vi "init.vi"(8 "error in (no error)":errorcluster, 11 "ILCTC in":refnum<class "ILCTC.lvclass">) -> (0 "error out":errorcluster, 3 "ILCTC out":refnum<class "ILCTC.lvclass">)   [LabVIEW 2015, in "ILCTC.lvclass"]
uses:
  ILCTC.lvclass
  <userlib>/Common/ILC/Configuration/Serial.ctl
  <userlib>/Common/SerialProtocols/Configuration/SerialConfig.ctl
  <userlib>/Common/SerialProtocols/Configuration/SerialProtocol.ctl
  <userlib>/Common/SerialProtocols/Configuration/ProtocolParameters.ctl
  <userlib>/Common/SerialProtocols/Configuration/SerialMessageParameters.ctl
  <userlib>/Common/ILC/Configuration/ADC Conversion Settings.ctl
  <userlib>/Common/ILC/Configuration/ADC Collection Settings.ctl
  <userlib>/Common/ILC/Typedefs/Input Channels.ctl
  <userlib>/Common/ILC/Typedefs/Scan Rates.ctl
  <userlib>/Common/ILC/Configuration/DAC Settings.ctl
  <userlib>/Common/ILC/ILC/ILC.lvclass/ILC.ctl
  <userlib>/Common/ILC/ILC/ILC.lvclass
  <userlib>/Common/SerialProtocols/SerialProtocols.lvlib
  <userlib>/Common/ILC/Configuration/ILCConfiguration.lvlib
  ConfigurationThisComponent/ConfigurationThisComponent.lvclass
  <userlib>/Common/ILC/Typedefs/ILCTypedefs.lvlib
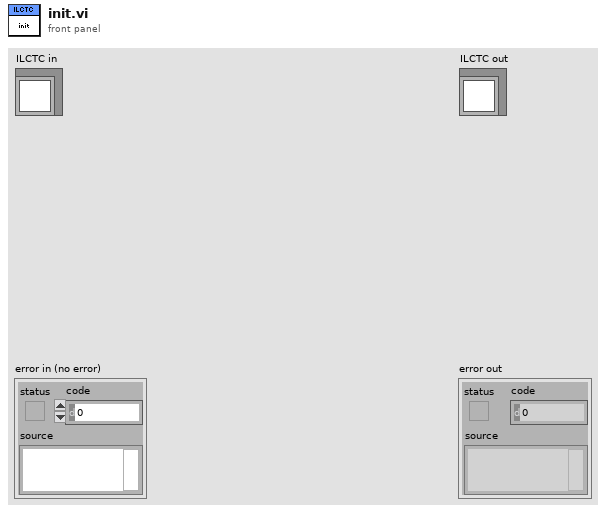
[diagram p1: front panel]
types:
  T1 = typedef "ILCCommon.lvlib/ILCConfiguration.lvlib/DAC Settings.ctl" = cluster{"Voltage Reference":dbl[unit], "Min Counts":i32, "Max Counts":i32}
  T2 = typedef "ILCCommon.lvlib/ILCConfiguration.lvlib/ADC Collection Settings.ctl" = cluster{"Input Channels":T3, "Scan Rate (Hz) ":T4, "PGA Gain Coefficient":u8}
  T3 = typedef "ILCCommon.lvlib/ILCTypedefs.lvlib/Input Channels.ctl" = enum16{"Channel 0", "3 Channels", "5 Channels"}
  T4 = typedef "ILCCommon.lvlib/ILCTypedefs.lvlib/Scan Rates.ctl" = enum16{"50", "60", "100", "120", "200", "240", "300", "400", "480", "600", "1200", "2400", "4800"}
  T5 = typedef "ILCCommon.lvlib/ILCConfiguration.lvlib/ADC Conversion Settings.ctl" = cluster{"Reference Voltage Vref":dbl[unit], "Nominal Input Range in Counts":u32, "Preamplifier Gain (K1 * K2)":dbl, "Conversion Settling Cycles":u16, "Excitation Voltage Vexc":dbl[unit]}
  T6 = typedef "ILCCommon.lvlib/ILCConfiguration.lvlib/Serial.ctl" = cluster{"Serial":T7}
  T7 = typedef "SerialProtocols.lvlib/SerialConfig.ctl" = cluster{"Serial Protocol":T8, "Protocol Parameters":T9, "Serial Message Parameters":T10}
  T8 = typedef "SerialProtocols.lvlib/SerialProtocol.ctl" = enum16{"RS232", "RS485", "SerialSimulator"}
  T9 = typedef "SerialProtocols.lvlib/ProtocolParameters.ctl" = cluster{"VISA resource name":refnum<visa-resource-name>, "Baud Rate":u32, "Data Bits":u16, "Parity":enum16{"None", "Odd", "Even", "Mark", "Space"}, "Flow Control":u16, "Stop Bits":u16, "Timeout (ms)":u32}
  T10 = typedef "SerialProtocols.lvlib/SerialMessageParameters.ctl" = cluster{"Byte Count":u32, "Enable Termination Character":bool, "Termination Char":u8}
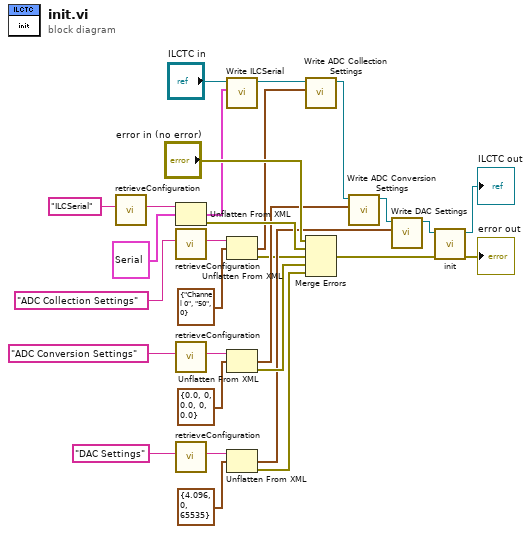
[diagram p0: block diagram]
diagram:
  n1 = call "retrieveConfiguration.vi"("configName"="ILCSerial") -> ("xmlConfig"=w24:string)  [unwired: 8 in, 2 out]
  n2 = Unflatten From XML(xml string=w24, type=T6 {"Serial"={"Serial Protocol"=enum."RS232", "Protocol Parameters"={"VISA resource name"="", "Baud Rate"=0, "Data Bits"=0, "Parity"=enum."None", "Flow Control"=0, "Stop Bits"=0, "Timeout (ms)"=0}, "Serial Message Parameters"={"Byte Count"=0, "Enable Termination Character"=FALSE, "Termination Char"=0}}} ("ILC")) -> (value=w18:T6, error out=w27:errorcluster)  [unwired: 1 in]
  n3 = call "retrieveConfiguration.vi"("configName"="ADC Collection Settings") -> ("xmlConfig"=w4:string)  [unwired: 8 in, 2 out]
  n4 = call "retrieveConfiguration.vi"("configName"="ADC Conversion Settings") -> ("xmlConfig"=w22:string)  [unwired: 8 in, 2 out]
  n5 = call "retrieveConfiguration.vi"("configName"="DAC Settings") -> ("xmlConfig"=w8:string)  [unwired: 8 in, 2 out]
  n6 = call <userlib>:"Write ILCSerial.vi"("ILC Serial"=w18, "ILC in"="ILCTC in") -> ("ILC out"=w12:refnum<class "ILCTC.lvclass">)  [unwired: 9 in]
  n7 = Unflatten From XML(xml string=w4, type=T2 {"Input Channels"=enum."Channel 0", "Scan Rate (Hz) "=enum."50", "PGA Gain Coefficient"=0} ("ADC Collection Settings")) -> (value=w2:T2, error out=w1:errorcluster)  [unwired: 1 in]
  n8 = Unflatten From XML(xml string=w22, type=T5 {"Reference Voltage Vref"=0.0, "Nominal Input Range in Counts"=0, "Preamplifier Gain (K1 * K2)"=0.0, "Conversion Settling Cycles"=0, "Excitation Voltage Vexc"=0.0} ("ILC ADC")) -> (value=w17:T5, error out=w21:errorcluster)  [unwired: 1 in]
  n9 = Unflatten From XML(xml string=w8, type=T1 {"Voltage Reference"=4.096, "Min Counts"=0, "Max Counts"=65535} ("DAC Settings")) -> (value=w6:T1, error out=w5:errorcluster)  [unwired: 1 in]
  n10 = call <userlib>:"Write ADC Collection Settings.vi"("ADC Collection Settings"=w2, "ILC in"=w12) -> ("ILC out"=w11:refnum<class "ILCTC.lvclass">)  [unwired: 9 in]
  n11 = Merge Errors("error in (no error)", w27, w1, w21, w5) -> (w16:errorcluster)
  n12 = call <userlib>:"Write ADC Conversion Settings.vi"("ADC Conversion Settings"=w17, "ILC in"=w11) -> ("ILC out"=w10:refnum<class "ILCTC.lvclass">)  [unwired: 9 in]
  n13 = call <userlib>:"Write DAC Settings.vi"("DAC Settings"=w6, "ILC in"=w10) -> ("ILC out"=w9:refnum<class "ILCTC.lvclass">)  [unwired: 9 in]
  n14 = call-parent "init.vi"("error in (no error)"=w16, "ILC in"=w9) -> ("error out"=→"error out":errorcluster, "ILC out"=→"ILCTC out":refnum<class "ILCTC.lvclass">)  [unwired: 8 in]
